vi "testtrigger.vi"() -> ()   [LabVIEW 2014]
uses:
  <vilib>/Utility/inputDevices.llb/joystickAcquire.vi
  <vilib>/Utility/inputDevices.llb/closeJoystick.vi
panel:
  out ".not. x?":bool
  out "llll":bool
  out "button 3":bool
  out "trap 1":bool
  in  "stop":bool
  out "button info":T1
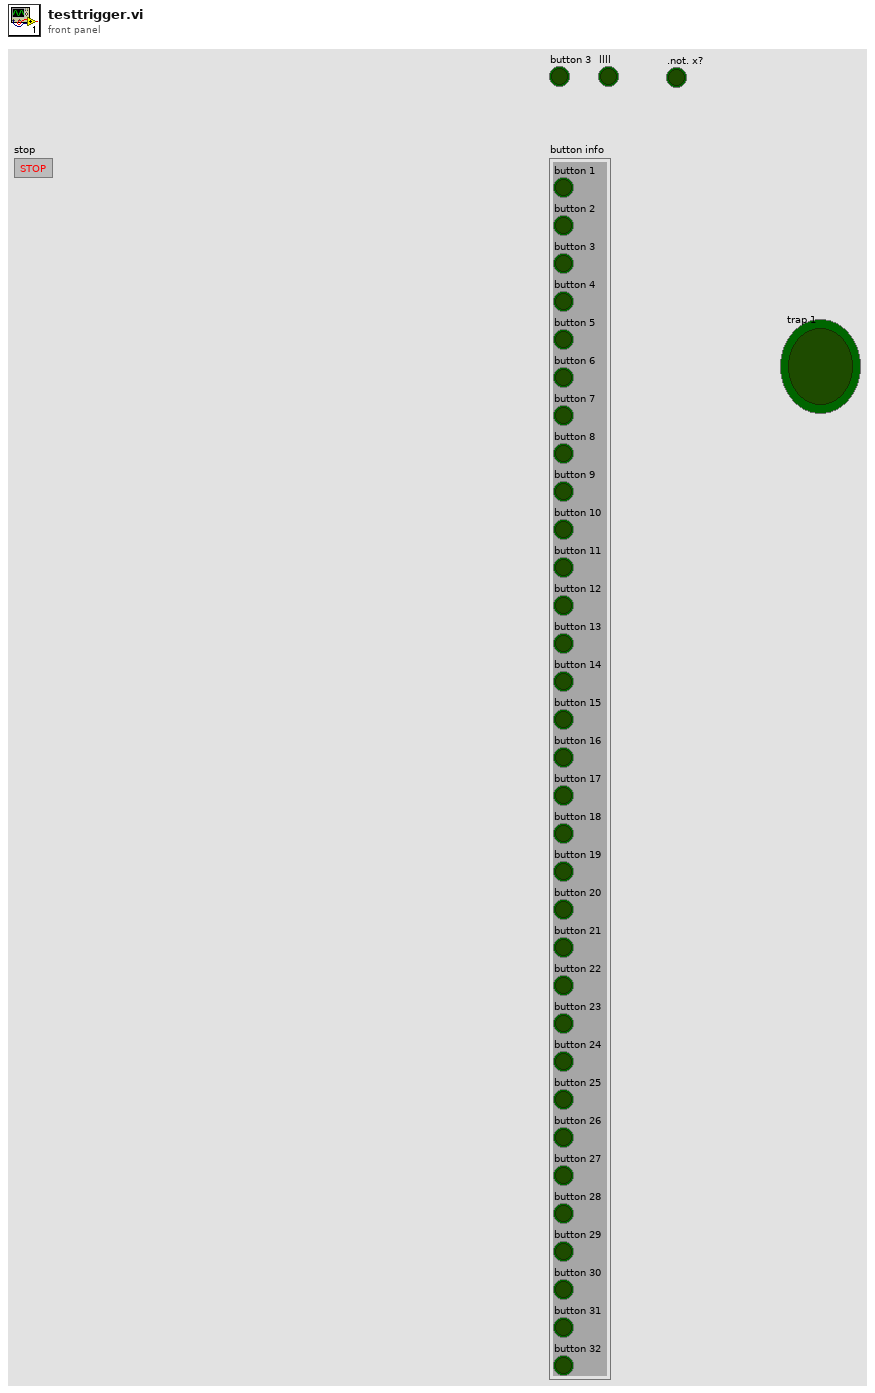
[diagram p1: front panel]
types:
  T1 = cluster{"button 1":bool, "button 2":bool, "button 3":bool, "button 4":bool, "button 5":bool, "button 6":bool, "button 7":bool, "button 8":bool, "button 9":bool, "button 10":bool, "button 11":bool, "button 12":bool, "button 13":bool, "button 14":bool, "button 15":bool, "button 16":bool, "button 17":bool, "button 18":bool, "button 19":bool, "button 20":bool, "button 21":bool, "button 22":bool, "button 23":bool, "button 24":bool, "button 25":bool, "button 26":bool, "button 27":bool, "button 28":bool, "button 29":bool, "button 30":bool, "button 31":bool, "button 32":bool}
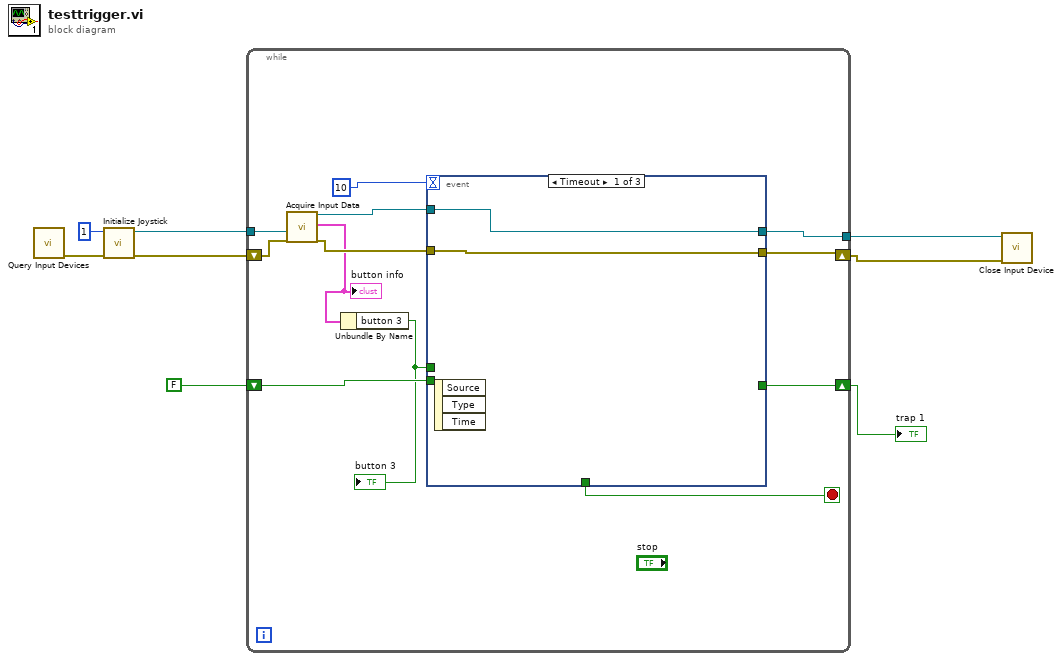
[diagram p0: block diagram]
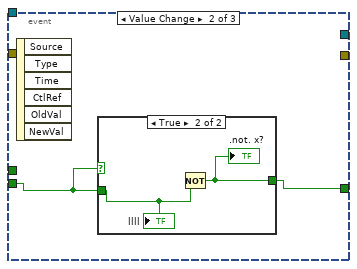
[diagram p2: hidden frame]
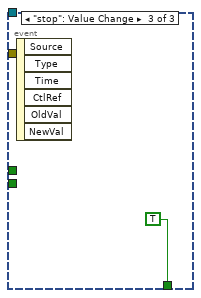
[diagram p4: hidden frame]
diagram:
  n1 = call <vilib>:"Query Input Devices.vi"() -> ("error out"=w7:errorcluster)  [unwired: 8 in, 3 out]
  n2 = call <vilib>:"Initialize Joystick.vi"("error in (no error)"=w7, "device index"=1) -> ("error out"=w6:errorcluster, "device ID"=w5:refnum<k1>)  [unwired: 8 in]
  n3 = while {
    tunnel: w5 -> [w17]
    tunnel: [w20] -> w4
    shift-right: [w19] -> w3
    shift-left: w6 -> [w16]
    shift-right: [w11] -> w1
    shift-left: FALSE ("button 3") -> [w18]
    stop <- w10 stop-if-true
    n4 = call-poly <vilib>:"Acquire Input Data.vi"("device ID"=w17, "error in (no error)"=w16) -> ("device ID 2"=w15:refnum<k1>, "button info"=w13:T1, "error out"=w14:errorcluster)  [unwired: 13 in, 2 out]
    "button info" <- w13
    n5 = Unbundle By Name(w13) -> ("button 3"=w12:bool)
    "button 3" <- w12
    n6 = event shown="[0] Timeout" {
      selector: _ -> [_ _ _]
      dyn-events: _ -> [_ _ _]
      timeout: 10 -> [_ _ _]
      tunnel: w14 -> [w21 _ _]
      tunnel: [w22 _ _] -> w20
      tunnel: [w21 _ _] -> w19
      tunnel: w18 -> [_ w23 _]
      tunnel: w15 -> [w22 _ _]
      tunnel: w12 -> [_ _ _]
      tunnel: [_ w24 _] -> w11
      tunnel: [_ _ TRUE ("button 3")] -> w10
      event Timeout {
        n7 = event-data() -> ()  [unwired: 1 in, 3 out]
      }
      event "button info.button 3": Value Change {
        n8 = event-data() -> ()  [unwired: 1 in, 6 out]
        n9 = case shown="True" w23 {
          tunnel: [w25 w26] -> w24
          tunnel: w23 -> [w25 w27]
          frame False {
          }
          frame True {
            n10 = Not(x=w27) -> (.not. x?=w26:bool)
            ".not. x?" <- w26
            "llll" <- w27
          }
        }
      }
      event "stop": Value Change {
        n11 = event-data() -> ()  [unwired: 1 in, 6 out]
      }
    }
  }
  "trap 1" <- w1
  n12 = call-poly <vilib>:"Close Input Device.vi"("error in (no error)"=w3, "device ID"=w4) -> ()  [unwired: 8 in, 1 out]
